vi "Configure Reference Channel (VBW and RBW).vi"(0 "VISA resource name":refnum<visa-resource-name>, 1 "Auto VBW/RBW Ratio (T: Enable)":bool=TRUE, 2 "Auto Resolution Bandwidth (T: Enable)":bool=TRUE, 3 "Auto Video Bandwidth (T: Enable)":bool=TRUE, 5 "Device Mode (1: BTS)":i32(ring)=1 items=["BTS"=1, "MS"=2], 11 "error in (no error)":errorcluster, 12 "Manual VBW/RBW Ratio (1)":dbl=1.0, 13 "Manual Resolution Bandwidth (3E+6 Hz)":i32=3000000, 14 "Manual Video Bandwidth (3E+6 Hz)":i32=3000000) -> (4 "VISA resource name out":refnum<visa-resource-name>, 15 "error out":errorcluster)   [LabVIEW 2018, in "Agilent MXA Series.lvlib"]
doc: "Configures the VBW and RWB settings of the reference channel in the Spectrumn Emission Mask measurement."
uses:
  Agilent MXA Series.lvlib
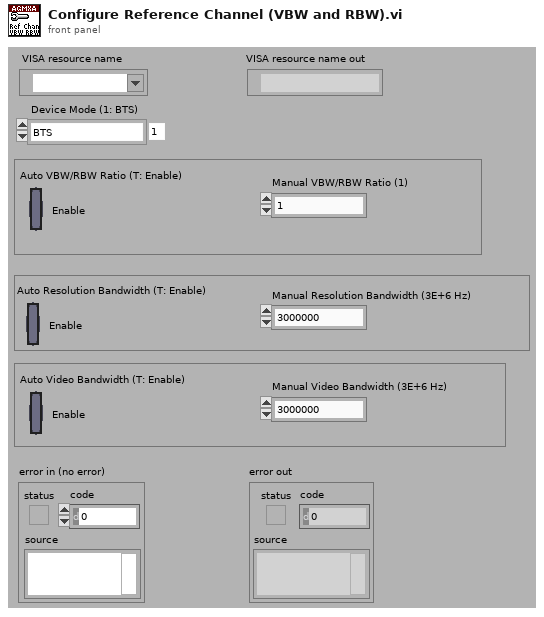
[diagram p1: front panel]
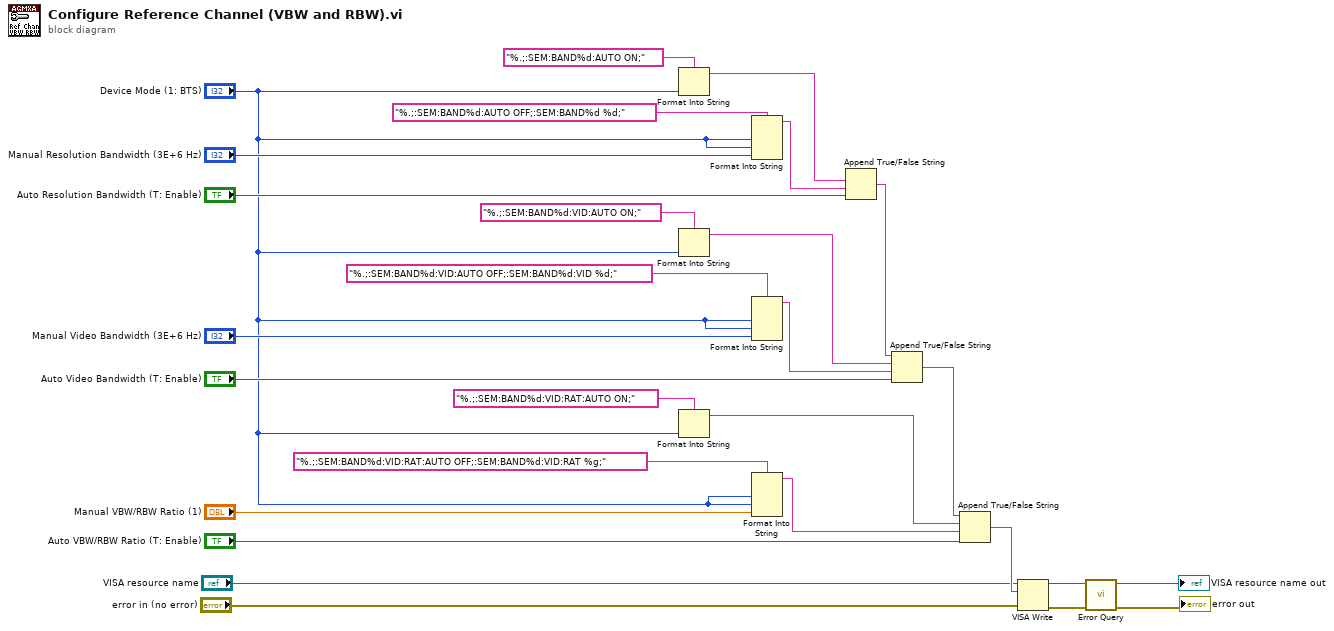
[diagram p0: block diagram]
diagram:
  n1 = Format Into String(format string="%.;:SEM:BAND%d:AUTO ON;" ("initial string"), "Device Mode (1: BTS)") -> (resulting string=w26:string)  [unwired: 2 in, 1 out]
  n2 = Format Into String(format string="%.;:SEM:BAND%d:VID:AUTO ON;" ("initial string"), "Device Mode (1: BTS)") -> (resulting string=w18:string)  [unwired: 2 in, 1 out]
  n3 = Format Into String(format string="%.;:SEM:BAND%d:VID:RAT:AUTO ON;", "Device Mode (1: BTS)") -> (resulting string=w10:string)  [unwired: 2 in, 1 out]
  n4 = Format Into String(format string="%.;:SEM:BAND%d:AUTO OFF;:SEM:BAND%d %d;" ("initial string"), "Device Mode (1: BTS)", "Device Mode (1: BTS)", "Manual Resolution Bandwidth (3E+6 Hz)") -> (resulting string=w27:string)  [unwired: 2 in, 1 out]
  n5 = Format Into String(format string="%.;:SEM:BAND%d:VID:AUTO OFF;:SEM:BAND%d:VID %d;" ("initial string"), "Device Mode (1: BTS)", "Device Mode (1: BTS)", "Manual Video Bandwidth (3E+6 Hz)") -> (resulting string=w17:string)  [unwired: 2 in, 1 out]
  n6 = Format Into String(format string="%.;:SEM:BAND%d:VID:RAT:AUTO OFF;:SEM:BAND%d:VID:RAT %g;" ("initial string"), "Device Mode (1: BTS)", "Device Mode (1: BTS)", "Manual VBW/RBW Ratio (1)") -> (resulting string=w9:string)  [unwired: 2 in, 1 out]
  n7 = Append True/False String(1:"Auto Resolution Bandwidth (T: Enable)", 2:w27, 3:w26) -> (0:w19:string)  [unwired: 1 in]
  n8 = Append True/False String(1:"Auto Video Bandwidth (T: Enable)", 2:w17, 3:w18, 4:w19) -> (0:w11:string)
  n9 = Append True/False String(1:"Auto VBW/RBW Ratio (T: Enable)", 2:w9, 3:w10, 4:w11) -> (0:w5:string)
  n10 = VISA Write(VISA resource name="VISA resource name", write buffer=w5, error in (no error)="error in (no error)") -> (VISA resource name out=w6:refnum<visa-resource-name>, error out=w7:errorcluster)  [unwired: 1 out]
  n11 = call "Error Query.vi"("error in (no error)"=w7, "VISA resource name"=w6) -> ("error out"=→"error out":errorcluster, "VISA resource name out"=→"VISA resource name out":refnum<visa-resource-name>)  [unwired: 6 in, 2 out]
